vi "LogMessage.vi"(0 "Type":enum16{"Locks", "Warning"}(ring), 1 "Reactor Name":string, 2 "Log Entry":string, 3 "System JSON Queue":refnum<vi>, 4 "ID Number":i32, 5 "System Queue":refnum<vi>) -> ()   [LabVIEW 2022 SP3]
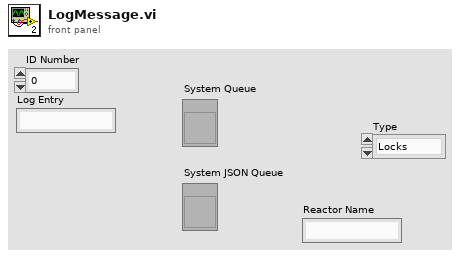
[diagram p1: front panel]
types:
  T1 = cluster{"LogMessage":string, "reactorName":string, "timeStamp":string}
  T2 = cluster{"type":string, "meta":string, "payload":cluster{"LogMessage":string, "reactorName":string, "timeStamp":string}}
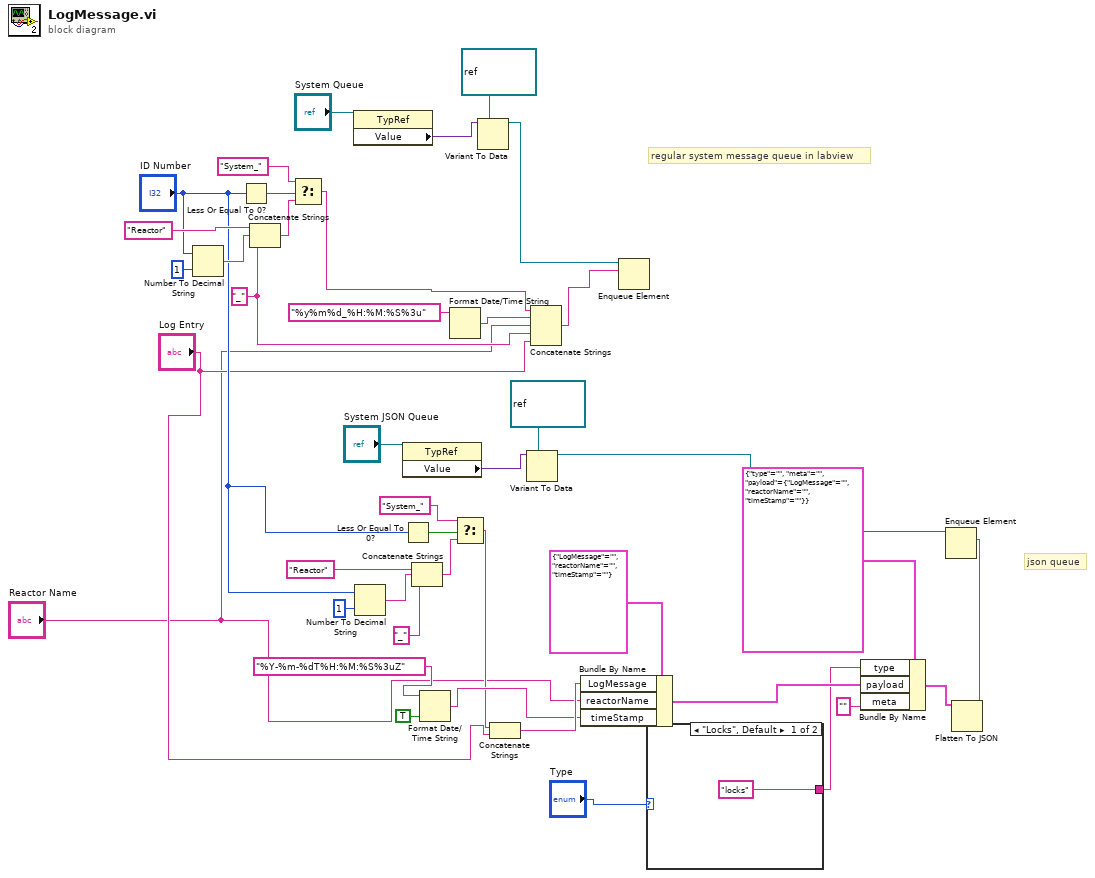
[diagram p0: block diagram]
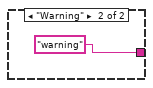
[diagram p2: hidden frame]
diagram:
  w2 = "_" ("string")
  # "json queue"
  # "regular system message queue in labview"
  n1 = Number To Decimal String(number="ID Number", width (-)=i16 1) -> (decimal integer string=w32:string)
  n2 = Less Or Equal To 0?(x="ID Number") -> (x <= 0?=w29:bool)
  n3 = Concatenate Strings("Reactor" ("string"), w32, w2) -> (w31:string)
  n4 = Select(t="System_" ("string"), s=w29, f=w31) -> (s? t:f=w30:string)
  n5 = property class="TypRef"(reference="System Queue") -> ("Value"=w37:variant)  [unwired: 1 in, 2 out]
  n6 = Number To Decimal String(number="ID Number", width (-)=i16 1) -> (decimal integer string=w23:string)
  n7 = property class="TypRef"(reference="System JSON Queue") -> ("Value"=w26:variant)  [unwired: 1 in, 2 out]
  n8 = Less Or Equal To 0?(x="ID Number") -> (x <= 0?=w21:bool)
  n9 = Concatenate Strings("Reactor" ("string"), w23, "_" ("string")) -> (w22:string)
  n10 = Format Date/Time String(time format string (%c)="%Y-%m-%dT%H:%M:%S%3uZ", UTC format=TRUE) -> (date/time string=w5:string)  [unwired: 1 in]
  n11 = Format Date/Time String(time format string (%c)="%y%m%d_%H:%M:%S%3u") -> (date/time string=w41:string)  [unwired: 2 in]
  n12 = Select(t="System_" ("string"), s=w21, f=w22) -> (s? t:f=w4:string)
  n13 = Variant To Data(type=refnum<queue> refnum ("Queue Reactor 6"), Variant=w37) -> (data=w36:refnum<queue>)  [unwired: 1 in, 1 out]
  n14 = Concatenate Strings(w4, "Log Entry") -> (w12:string)
  n15 = Variant To Data(type=refnum<queue> refnum ("Queue Reactor 6"), Variant=w26) -> (data=w25:refnum<queue>)  [unwired: 1 in, 1 out]
  n16 = Concatenate Strings(w30, w41, "Reactor Name", w2, "Log Entry") -> (w40:string)
  n17 = Bundle By Name(cluster=T1 {"LogMessage"="", "reactorName"="", "timeStamp"=""} ("input cluster"), "LogMessage"=w12, "reactorName"="Reactor Name", "timeStamp"=w5) -> (w16:T1)
  n18 = Enqueue Element(queue=w36, element=w40) -> ()  [unwired: 2 in, 3 out]
  n19 = case shown="\"Locks\", Default" "Type" {
    tunnel: ["locks" "warning"] -> w8
    frame "Locks", Default {
    }
    frame "Warning" {
    }
  }
  n20 = Bundle By Name(cluster=T2 {"type"="", "meta"="", "payload"={"LogMessage"="", "reactorName"="", "timeStamp"=""}} ("input cluster"), "type"=w8, "payload"=w16, "meta"="") -> (w7:T2)
  n21 = Flatten To JSON(anything=w7) -> (JSON string=w6:string)  [unwired: 2 in, 1 out]
  n22 = Enqueue Element(queue=w25, element=w6) -> ()  [unwired: 2 in, 3 out]
